vi "Vision Processing (3).vi"(4 "Error In":errorcluster, 7 "Image Size":T4=enum."320x240") -> ()   [LabVIEW 2016]
doc: "This VI runs in parallel to other tasks. It gets images from the camera, processes them for color or shape and use that information to affect robot behavior."
uses:
  <vilib>/Rock Robotics/WPI/Camera/WPI_CameraImageSize.ctl
  <vilib>/Rock Robotics/WPI/Camera/WPI_CameraWhite Balance Values.ctl
  <vilib>/Rock Robotics/WPI/Camera/WPI_CameraExposure Values.ctl
  <vilib>/Rock Robotics/WPI/Camera/WPI_CameraFrameRate.ctl
  Robot Global Data.vi
panel:
  in  "R/G/B":cluster{"Lower value":i32, "Upper value":i32}[](array[cluster])=[{"Lower value"=0, "Upper value"=200}, {"Lower value"=230, "Upper value"=255}, {"Lower value"=210, "Upper value"=255}]
  out "New Image":T1(plugin-control)
  out "Bounding Box Final":T2
  out "Particle Report 2":T3
  out "Particle Report":T3
  out "Thresholded Image":T1(plugin-control)
  out "Error Out":errorcluster
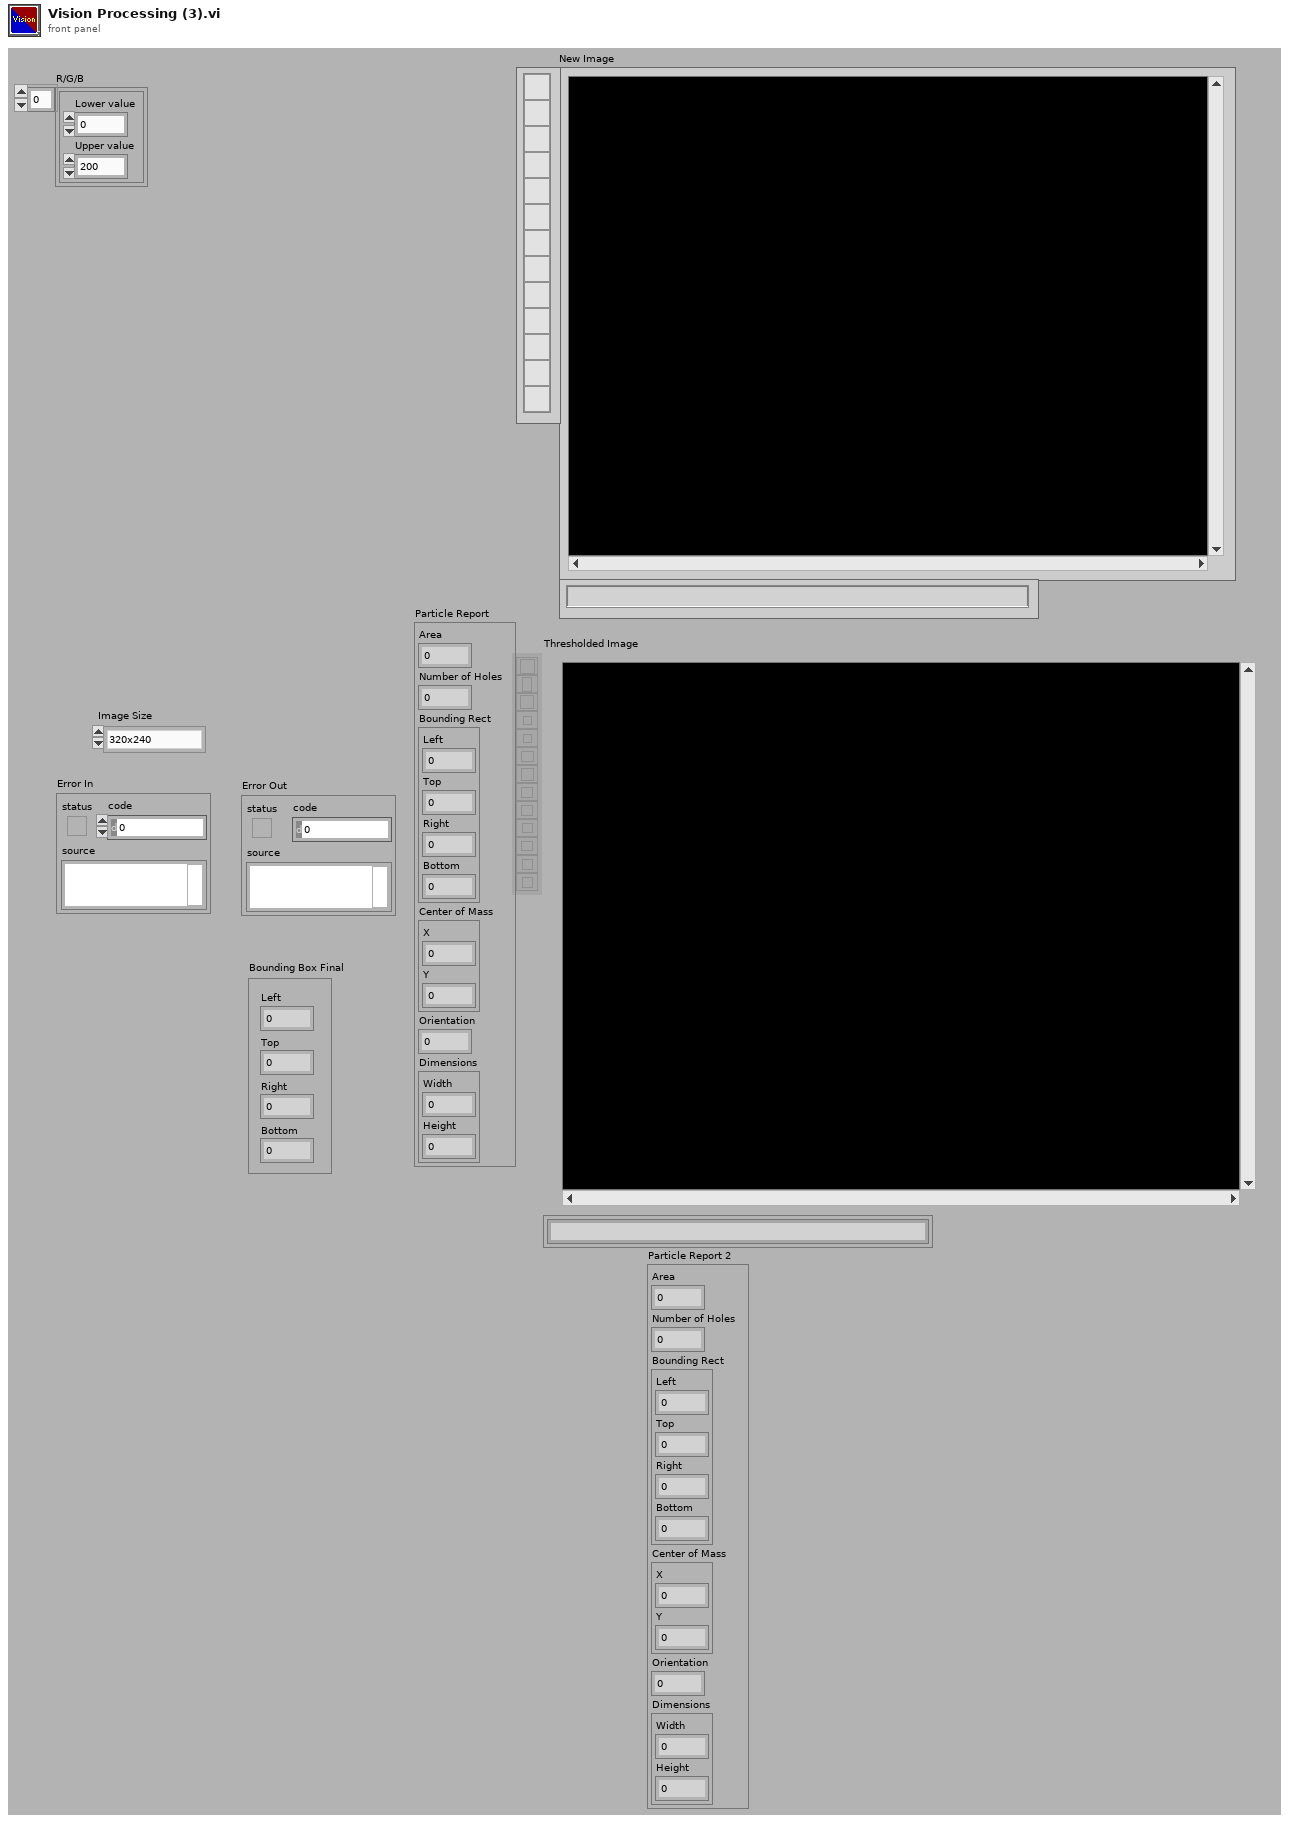
[diagram p1: front panel]
types:
  T1 = typedef "IMAQ Image.ctl" = refnum<image>
  T2 = cluster{"Left":dbl, "Top":dbl, "Right":dbl, "Bottom":dbl}
  T3 = cluster{"Area":dbl, "Number of Holes":dbl, "Bounding Rect":cluster{"Left":dbl, "Top":dbl, "Right":dbl, "Bottom":dbl}, "Center of Mass":cluster{"X":dbl, "Y":dbl}, "Orientation":dbl, "Dimensions":cluster{"Width":dbl, "Height":dbl}}
  T4 = typedef "WPI_CameraImageSize.ctl" = enum16{"640x480", "320x240", "160x120", "Custom"}
  T5 = typedef "Image Type" = u32
  T6 = typedef "WPI_CameraFrameRate.ctl" = u32
  T7 = typedef "WPI_CameraExposure Values.ctl" = enum16{"Auto", "Flicker-free 50 Hz", "Flicker-free 60 Hz", "Hold current", "Custom"}
  T8 = typedef "WPI_CameraWhite Balance Values.ctl" = enum16{"Auto", "Fixed indoor", "Fixed outdoor 1", "Fixed outdoor 2", "Fixed fluorescent 1", "Fixed fluorescent 2", "Hold current", "Custom"}
  T9 = typedef "WPI_CameraDevRef.ctl" = cluster{"Camera Address":string, "CameraStatus":errorcluster}
  T10 = cluster{"Bounding Box Final":cluster{"Left":dbl, "Top":dbl, "Right":dbl, "Bottom":dbl}, "X Resolution":i32, "Y Resolution":i32}
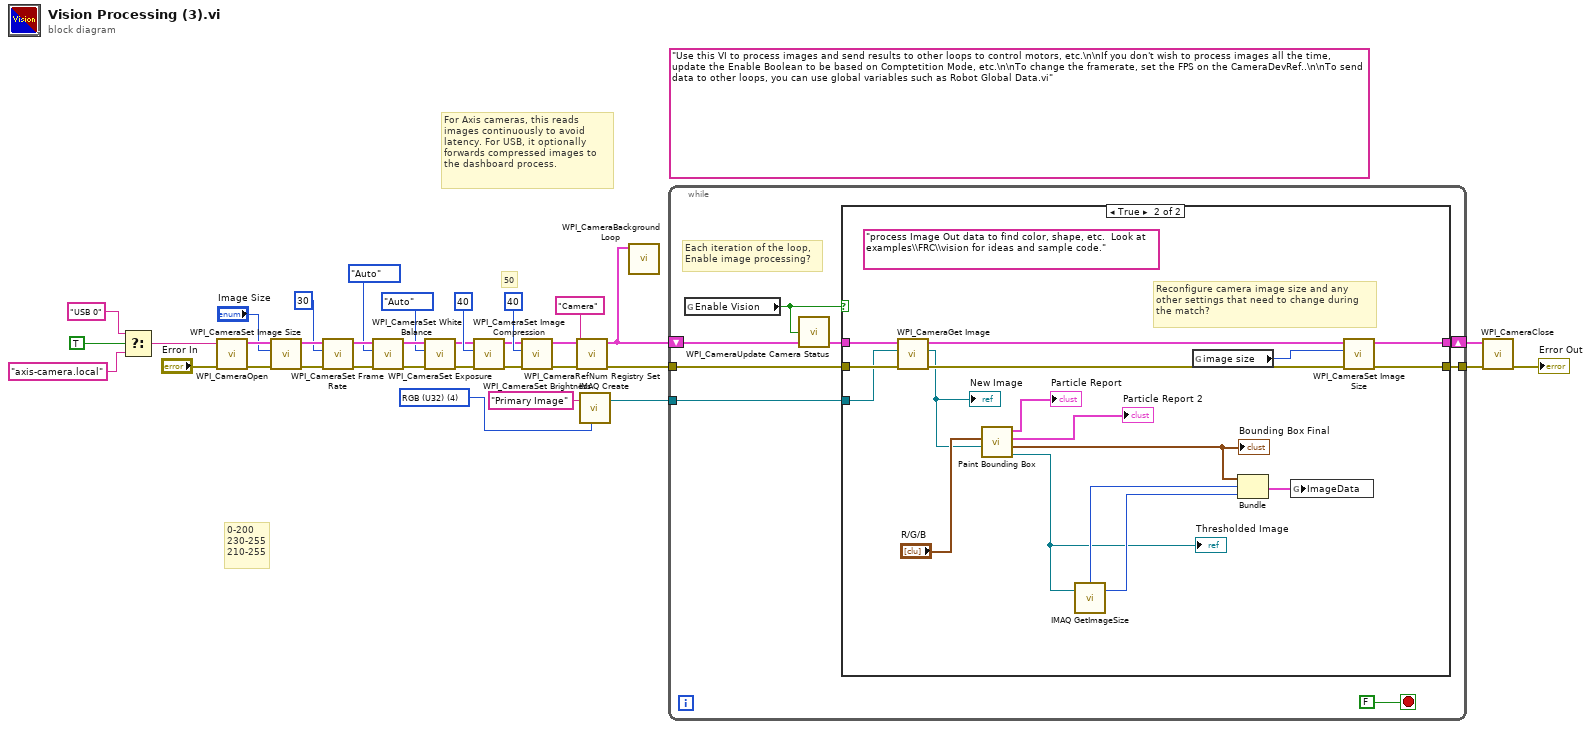
[diagram p0: block diagram]
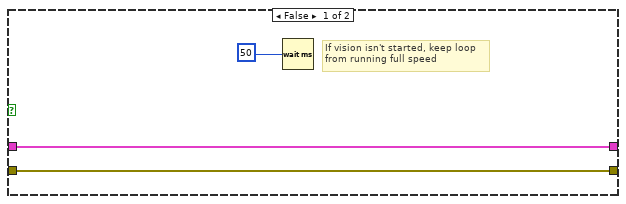
[diagram p2: hidden frame]
diagram:
  w5 = T5 4 items=["Grayscale (U8)", "Grayscale (I16)", "Grayscale (SGL)", "Complex (CSG)", "RGB (U32)", "HSL (U32)", "RGB (U64)"] ("Image Type")
  (unwired) "Use this VI to process images and send results to other loops to control motors, etc.\n\nIf you don't wish to process images all the time, update the Enable Boolean to be based on Comptetition Mode, etc.\n\nTo change the framerate, set the FPS on the CameraDevRef..\n\nTo send data to other loops, you can use global variables such as Robot Global Data.vi"
  # "0-200\n230-255\n210-255"
  # "50"
  # "For Axis cameras, this reads\nimages continuously to avoid\nlatency. For USB, it optionally\nforwards compressed images to\nthe dashboard process."
  n1 = Select(t="USB 0" ("format string"), s=TRUE ("dot notation? (F)"), f="axis-camera.local" ("format string")) -> (s? t:f=w8:string)
  n2 = call <vilib>:"WPI_CameraOpen.vi"("error in (no error)"="Error In", "Camera Address"=w8) -> ("error out"=w24:errorcluster, "CameraDevRef"=w25:T9)  [unwired: 8 out]
  n3 = call <vilib>:"WPI_CameraSet Image Size.vi"("error in (no error)"=w24, "Image Size"="Image Size", "CameraDevRef"=w25) -> ("error out"=w23:errorcluster, "CameraDevRef Out"=w26:T9)  [unwired: 1 in, 6 out]
  n4 = call <vilib>:"WPI_CameraSet Frame Rate.vi"("error in (no error)"=w23, "Frame Rate (fps)"=T6 30, "CameraDevRef"=w26) -> ("error out"=w22:errorcluster, "CameraDevRef Out"=w28:T9)  [unwired: 7 out]
  n5 = call <vilib>:"WPI_CameraSet White Balance.vi"("error in (no error)"=w22, "White Balance"=WPI_CameraWhite_Balance_Values."Auto", "CameraDevRef"=w28) -> ("error out"=w21:errorcluster, "CameraDevRef Out"=w27:T9)  [unwired: 1 in, 6 out]
  n6 = call <vilib>:"WPI_CameraSet Exposure.vi"("error in (no error)"=w21, "Exposure"=WPI_CameraExposure_Values."Auto", "CameraDevRef"=w27) -> ("error out"=w20:errorcluster, "CameraDevRef Out"=w30:T9)  [unwired: 1 in, 6 out]
  n7 = call <vilib>:"WPI_CameraSet Image Compression.vi"("error in (no error)"=w20, "Compression"=40, "CameraDevRef"=w30) -> ("error out"=w19:errorcluster, "CameraDevRef Out"=w29:T9)  [unwired: 7 out]
  n8 = call <vilib>:"WPI_CameraSet Brightness.vi"("error in (no error)"=w19, "Brightness"=40, "CameraDevRef"=w29) -> ("error out"=w17:errorcluster, "CameraDevRef Out"=w18:T9)  [unwired: 7 out]
  n9 = call <vilib>:"WPI_CameraRefNum Registry Set.vi"("error in (no error)"=w17, "refnum name"="Camera", "CameraDevRef"=w18) -> ("error out"=w1:errorcluster, "CameraDevRef"=w13:T9)  [unwired: 1 in, 6 out]
  n10 = call "IMAQ Create"("Image Name"="Primary Image", "Image Type"=w5) -> ("New Image"=w34:T1)  [unwired: 2 in, 2 out]
  n11 = call <vilib>:"WPI_CameraBackground Loop.vi"("CameraDevRef"=w13) -> ()  [unwired: 11 in]
  n12 = while {
    shift-right: [w41] -> w11
    shift-left: w13 -> [w39]
    tunnel: w34 -> [w40]
    tunnel: [w36] -> w2
    tunnel: w1 -> [w35]
    stop <- FALSE stop-if-true
    # "Each iteration of the loop,\nEnable image processing?"
    n13 = global read "Robot Global Data.vi" "Enable Vision"() -> (w37:bool)
    n14 = call <vilib>:"WPI_CameraUpdate Camera Status.vi"("CameraDevRef In"=w39, "Enable Vision"=w37) -> ("CameraDevRef Out"=w38:T9)  [unwired: 3 in]
    n15 = case shown="True" w37 {
      tunnel: w40 -> [_ w55]
      tunnel: [w45 w62] -> w41
      tunnel: w38 -> [w45 w60]
      tunnel: [w43 w58] -> w36
      tunnel: w35 -> [w43 w57]
      frame False {
        # "If vision isn't started, keep loop\nfrom running full speed"
        n16 = Wait (ms)(milliseconds to wait=u32 50) -> ()  [unwired: 1 out]
      }
      frame True {
        (unwired) "process Image Out data to find color, shape, etc.  Look at examples\\FRC\\vision for ideas and sample code."
        # "Reconfigure camera image size and any\nother settings that need to change during\nthe match?"
        n17 = call <vilib>:"WPI_CameraGet Image.vi"("error in (no error)"=w57, "Image"=w55, "CameraDevRef"=w60) -> ("error out"=w56:errorcluster, "Image Out"=w46:T1, "CameraDevRef Out"=w59:T9)  [unwired: 6 out]
        "New Image" <- w46
        n18 = call "Paint Bounding Box.vi"("Camera Image"=w46, "R/G/B"="R/G/B") -> ("Thresholded Image"=w47:T1, "Bounding Box Final"=w51:T2, "Particle Report 2"=→"Particle Report 2":T3, "Particle Report"=→"Particle Report":T3)  [unwired: 5 in, 1 out]
        "Thresholded Image" <- w47
        "Bounding Box Final" <- w51
        n19 = call "IMAQ GetImageSize"("Image"=w47) -> ("Y Resolution"=w49:i32, "X Resolution"=w50:i32)  [unwired: 3 in, 1 out]
        n20 = global read "Robot Global Data.vi" "image size"() -> (w61:T4)
        n21 = Bundle("Bounding Box Final"=w51, "X Resolution"=w50, "Y Resolution"=w49) -> (w48:T10)  [unwired: 1 in]
        n22 = global write "Robot Global Data.vi" "ImageData"(w48) -> ()
        n23 = call <vilib>:"WPI_CameraSet Image Size.vi"("error in (no error)"=w56, "Image Size"=w61, "CameraDevRef"=w59) -> ("error out"=w58:errorcluster, "CameraDevRef Out"=w62:T9)  [unwired: 1 in, 6 out]
      }
    }
  }
  n24 = call <vilib>:"WPI_CameraClose.vi"("error in (no error)"=w2, "CameraDevRef"=w11) -> ("error out"=→"Error Out":errorcluster)  [unwired: 9 out]
